vi "Teleop.vi"(10 "Match Info":T1={"Autonomous Elapsed Seconds"=0.0, "TeleOp Elapsed Seconds"=0.0, "Disabled Elapsed Seconds"=0.0, "Visited Autonomous"=FALSE, "Visited TeleOp"=FALSE, "Visited Disabled"=FALSE, "Autonomous Settings"={"Autonomous Style"=enum."Independent", "VI Refnum"=refnum}}, 11 "Call Context":T2) -> ()   [LabVIEW 2019]
doc: "This VI is called for each TeleOp packet received from the DS where the robot is not disabled. It is often used to read from the joysticks and update I/O or to update setpoints for timed control loops. It should complete and return within 20 milliseconds or it may miss DS packets."
uses:
  <vilib>/Rock Robotics/WPI/DriverStation/WPI_DriverStationDerivedRobotMode.ctl
  <vilib>/Rock Robotics/WPI/DriverStation/WPI_DriverStationMatch Info.ctl
  <vilib>/Rock Robotics/WPI/Solenoid/WPI_SolenoidValue.ctl
  <vilib>/Rock Robotics/WPI/ThirdParty/Phoenix-LabVIEW/Motor Controller/Controls/CTRE_Phoenix_MotorControl_ControlMode.ctl
  SubVi's/Joystick Organization/Joystick Global 6740.vi
  <vilib>/Rock Robotics/WPI/Solenoid/WPI_SolenoidSetEnum.vi
  <vilib>/Rock Robotics/WPI/ThirdParty/Phoenix-LabVIEW/Motor Controller/Get/CTRE_Phoenix_MotorController_GetSelectedSensorData.vi
  SubVi's/Global Conveyor.vi
panel:
  out "Color Count 2":dbl
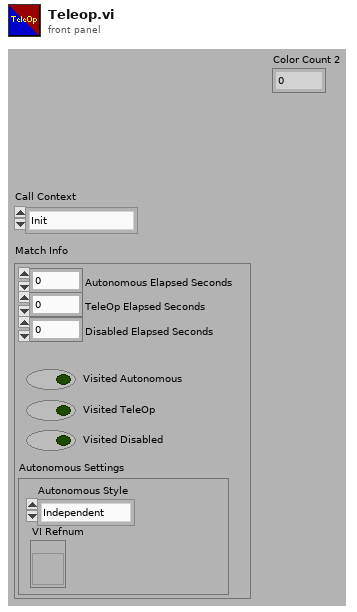
[diagram p1: front panel]
types:
  T1 = typedef "WPI_DriverStationMatch Info.ctl" = cluster{"Autonomous Elapsed Seconds":dbl, "TeleOp Elapsed Seconds":dbl, "Disabled Elapsed Seconds":dbl, "Visited Autonomous":bool, "Visited TeleOp":bool, "Visited Disabled":bool, "Autonomous Settings":cluster{"Autonomous Style":enum16{"Iterative", "Independent"}, "VI Refnum":refnum<vi>}}
  T2 = typedef "WPI_DriverStationDerivedRobotMode.ctl" = enum16{"Init", "Execute", "Stop"}
  T3 = typedef "WPI_SolenoidValue.ctl" = enum16{"Off", "On", "Forward", "Reverse"}
  T4 = typedef "WPI_MotorControlDeviceRef.ctl" = cluster{"DeviceStatus":errorcluster, "Type":T5, "PWM":cluster{"PWM Channel":T6, "DeadBand":T7}, "CAN":cluster{"Device Number":u8, "SetOutput VI Ref":variant, "GetOutput VI Ref":variant, "Enable VI Ref":variant, "Disable VI Ref":variant, "Data":variant}, "Invert":bool, "DIO PWM":cluster{"PWM \"Enable\" Channel":T6, "DIOChannel":T8, "PWM Rate":dbl}}
  T5 = typedef "WPI_MotorControlType.ctl" = enum16{"PWM", "CAN", "DIO PWM"}
  T6 = typedef "FPGA_DIOPWMChannel.ctl" = enum8{"PWM 0", "PWM 1", "PWM 2", "PWM 3", "PWM 4", "PWM 5", "PWM 6", "PWM 7", "PWM 8", "PWM 9", "PWM MXP 0", "PWM MXP 1", "PWM MXP 2", "PWM MXP 3", "PWM MXP 4", "PWM MXP 5", "PWM MXP 6", "PWM MXP 7", "PWM MXP 8", "PWM MXP 9", "Invalid"}
  T7 = typedef "WPI_PWMDeadband.ctl" = cluster{"Name":string, "maxPositivePwm":i32, "minPositivePwm":i32, "centerPwm":i32, "maxNegativePwm":i32, "minNegativePwm":i32, "angularRange":u16}
  T8 = typedef "FPGA_DIOChannel.ctl" = enum8{"DIO 0", "DIO 1", "DIO 2", "DIO 3", "DIO 4", "DIO 5", "DIO 6", "DIO 7", "DIO 8", "DIO 9", "DIO MXP 0", "DIO MXP 1", "DIO MXP 2", "DIO MXP 3", "DIO MXP 4", "DIO MXP 5", "DIO MXP 6", "DIO MXP 7", "DIO MXP 8", "DIO MXP 9", "DIO MXP 10", "DIO MXP 11", "DIO MXP 12", "DIO MXP 13", "DIO MXP 14", "DIO MXP 15", "SPI Port CS1", "SPI Port CS2", "SPI Port CS3", "SPI Port MISO", "SPI Port MOSI", "Invalid"}
  T9 = typedef "WPI_SolenoidDevRef.ctl" = cluster{"DevStatus":errorcluster, "Pneumatics Control Module":u8, "Forward Solenoid Channel":T10, "Reverse Solenoid Channel":T10}
  T10 = typedef "WPI_SolenoidChannel.ctl" = enum8{"Solenoid 0", "Solenoid 1", "Solenoid 2", "Solenoid 3", "Solenoid 4", "Solenoid 5", "Solenoid 6", "Solenoid 7", "Invalid"}
  T11 = typedef "Color Sensor V3 DevRef.ctl" = cluster{"I2CDevRef":T12}
  T12 = typedef "WPI_I2CDevRef.ctl" = cluster{"DevStatus":errorcluster, "Device Address":u8, "Handle":i32, "I2C Bus":T13}
  T13 = typedef "i2c_bus.ctl" = enum16{"I2C On-Board", "I2C MXP", "Invalid"}
  T14 = typedef "CTRE_Phoenix_MotorControl_ControlMode.ctl" = u16
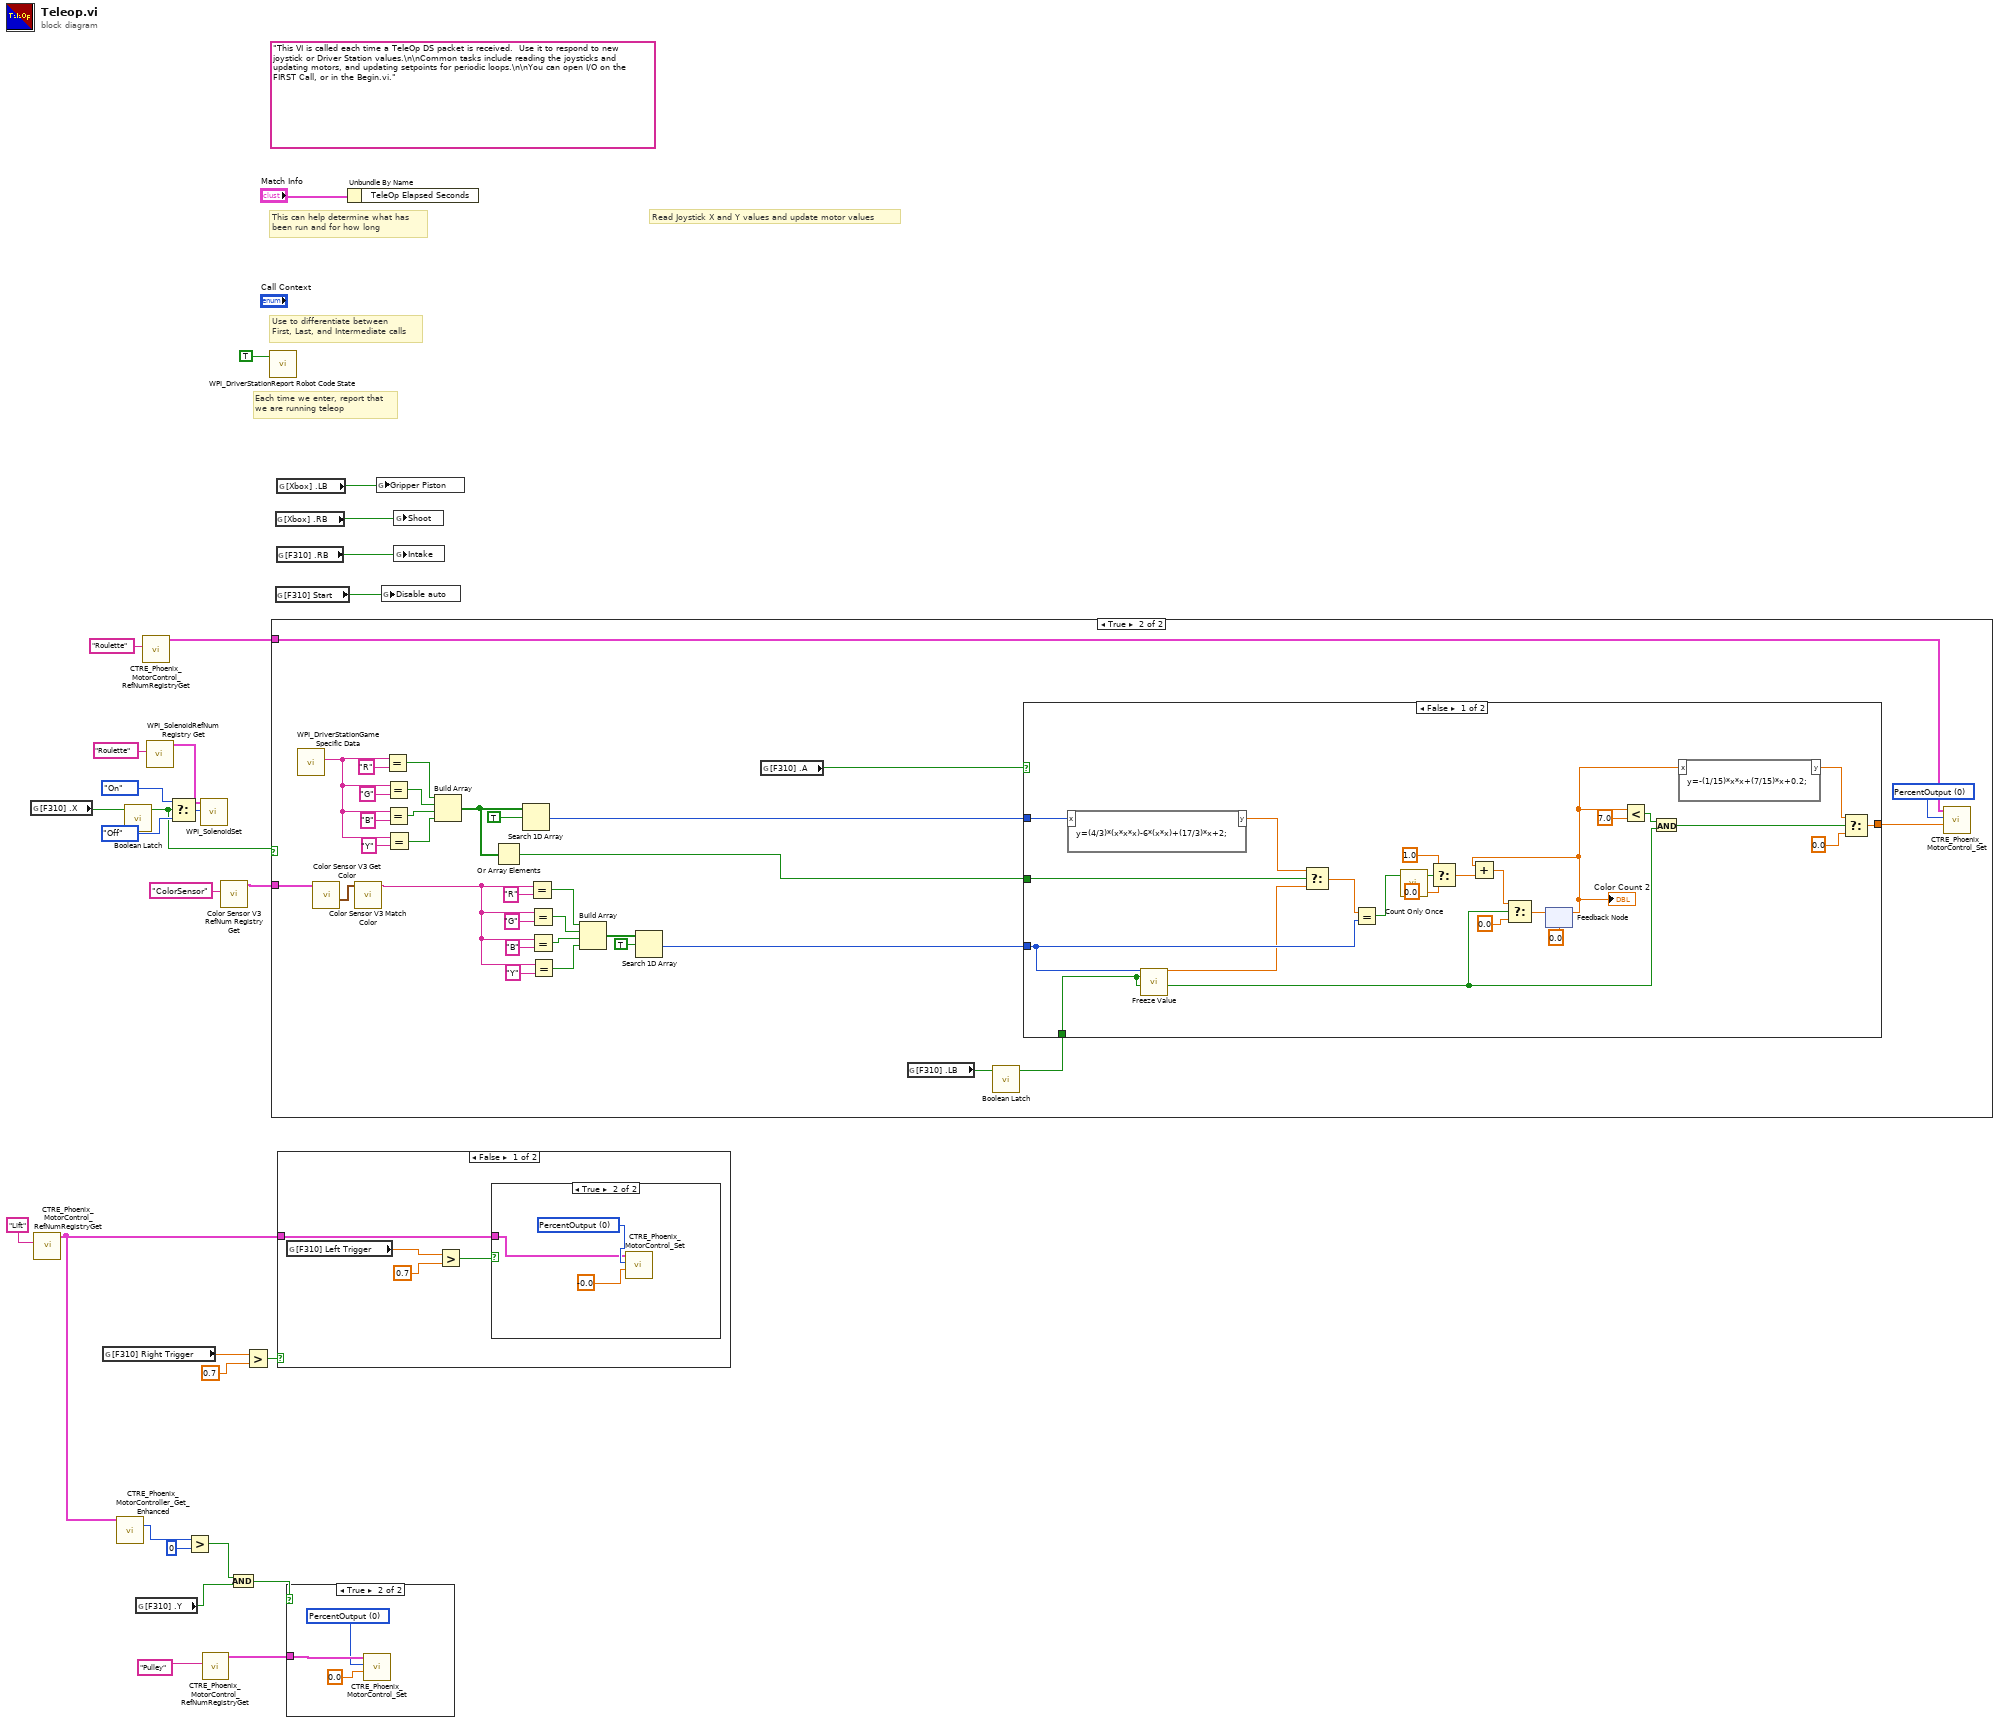
[diagram p0: block diagram]
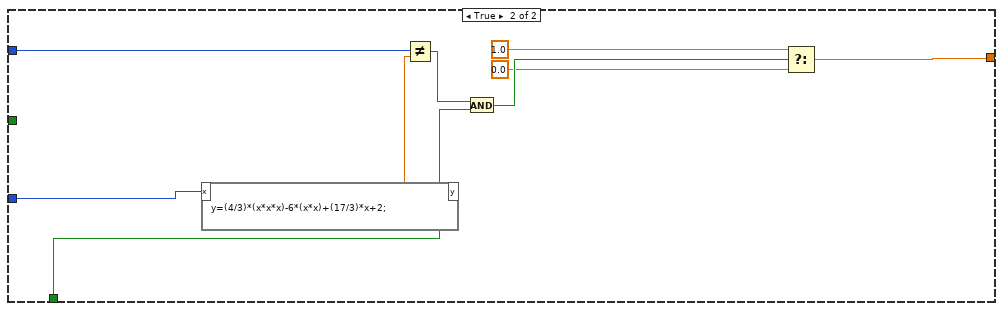
[diagram p3: hidden frame]
diagram:
  (unwired) "This VI is called each time a TeleOp DS packet is received.  Use it to respond to new joystick or Driver Station values.\n\nCommon tasks include reading the joysticks and updating motors, and updating setpoints for periodic loops.\n\nYou can open I/O on the FIRST Call, or in the Begin.vi."
  # "Each time we enter, report that\nwe are running teleop"
  # "Use to differentiate between\nFirst, Last, and Intermediate calls"
  # "This can help determine what has\nbeen run and for how long"
  # "Read Joystick X and Y values and update motor values"
  n1 = global read "Joystick Global 6740.vi" "[F310] .X"() -> (w13:bool)
  n2 = call <vilib>:"CTRE_Phoenix_MotorControl_RefNumRegistryGet.vi"("refnum name"="Lift") -> ("PhoenixMotorControlDevRef"=w23:T4)  [unwired: 9 in, 1 out]
  n3 = global read "Joystick Global 6740.vi" "[F310] Right Trigger"() -> (w27:dbl)
  n4 = call-poly <vilib>:"CTRE_Phoenix_MotorController_Get_Enhanced.vi"("PhoenixMotorControlDevRef"=w23) -> ("Position (Raw Sensor Units)"=w22:i32)  [unwired: 11 in, 3 out]
  n5 = call "Boolean Latch.vi"("Input"=w13) -> ("Output"=w7:bool)  [unwired: 26 in]
  n6 = global read "Joystick Global 6740.vi" "[F310] .Y"() -> (w19:bool)
  n7 = call <vilib>:"CTRE_Phoenix_MotorControl_RefNumRegistryGet.vi"("refnum name"="Roulette") -> ("PhoenixMotorControlDevRef"=w6:T4)  [unwired: 9 in, 1 out]
  n8 = call <vilib>:"WPI_SolenoidRefNum Registry Get.vi"("refnum name"="Roulette") -> ("SolenoidDevRef"=w14:T9)  [unwired: 9 in, 1 out]
  n9 = Select(t=WPI_SolenoidValue."On" ("Value"), s=w7, f=WPI_SolenoidValue."Off" ("Value")) -> (s? t:f=w10:T3)
  n10 = Greater?(x=w22, y=0) -> (0:w20:bool)
  n11 = call-poly <vilib>:"WPI_SolenoidSet.vi"("Value"=w10, "SolenoidDevRef"=w14) -> ()  [unwired: 8 in, 2 out]
  n12 = call <vilib>:"CTRE_Phoenix_MotorControl_RefNumRegistryGet.vi"("refnum name"="Pulley") -> ("PhoenixMotorControlDevRef"=w16:T4)  [unwired: 9 in, 1 out]
  n13 = call <vilib>:"Color Sensor V3 RefNum Registry Get.vi"("refnum name"="ColorSensor") -> ("ColorSensorDevRef"=w5:T11)  [unwired: 9 in, 1 out]
  n14 = And(x=w20, y=w19) -> (x .and. y?=w18:bool)
  n15 = Greater?(x=w27, y=0.7) -> (0:w25:bool)
  n16 = call <vilib>:"WPI_DriverStationReport Robot Code State.vi"("TeleOp"=TRUE ("Autonomous")) -> ()  [unwired: 10 in, 1 out]
  n17 = case shown="True" w7 {
    tunnel: w6 -> [_ w30]
    tunnel: w5 -> [_ w32]
    frame False {
    }
    frame True {
      w38 = T14 0 items=["PercentOutput"=0, "Position"=1, "Velocity"=2, "Current"=3, "Follower"=5, "MotionProfile"=6, "MotionMagic"=7, "MotionProfileArc"=10, "Disabled"=15] ("Control Mode")
      n18 = call <vilib>:"WPI_DriverStationGame Specific Data.vi"() -> ("Game Specific Data"=w35:string)  [unwired: 11 in]
      n19 = call <vilib>:"Color Sensor V3 Get Color.vi"("ColorSensorDevRef"=w32) -> ("Normalized Color"=w34:cluster{"R":dbl, "G":dbl, "B":dbl})  [unwired: 7 in, 3 out]
      n20 = call <vilib>:"Color Sensor V3 Match Color.vi"("Measured Color"=w34) -> ("Matched Color Name"=w33:string)  [unwired: 8 in, 2 out]
      n21 = Equal?(x=w35, y="R") -> (x = y?=w58:bool)
      n22 = Equal?(x=w35, y="G") -> (x = y?=w57:bool)
      n23 = Equal?(x=w35, y="B") -> (x = y?=w56:bool)
      n24 = Equal?(x=w35, y="Y") -> (x = y?=w55:bool)
      n25 = Build Array(w58, w57, w56, w55) -> (w42:bool[])
      n26 = Or Array Elements(Boolean array=w42) -> (logical OR=w40:bool)
      n27 = Search 1D Array(1D array=w42, element=TRUE) -> (index of element=w41:i32)  [unwired: 1 in]
      n28 = Equal?(x=w33, y="R") -> (x = y?=w52:bool)
      n29 = Equal?(x=w33, y="G") -> (x = y?=w51:bool)
      n30 = Equal?(x=w33, y="B") -> (x = y?=w50:bool)
      n31 = Equal?(x=w33, y="Y") -> (x = y?=w49:bool)
      n32 = Build Array(w52, w51, w50, w49) -> (w53:bool[])
      n33 = Search 1D Array(1D array=w53, element=TRUE) -> (index of element=w39:i32)  [unwired: 1 in]
      n34 = global read "Joystick Global 6740.vi" "[F310] .A"() -> (w36:bool)
      n35 = global read "Joystick Global 6740.vi" "[F310] .LB"() -> (w31:bool)
      n36 = call "Boolean Latch.vi"("Input"=w31) -> ("Output"=w43:bool)  [unwired: 26 in]
      n37 = case shown="False" w36 {
        tunnel: w41 -> [w85 w94]
        tunnel: w43 -> [w68 w92]
        tunnel: [w70 w89] -> w37
        tunnel: w40 -> [w67 _]
        tunnel: w39 -> [w84 w91]
        frame False {
          n38 = formula code="y=(4/3)*(x*x*x)-6*(x*x)+(17/3)*x+2;"("x"=w85) -> ("y"=w78:dbl)
          n39 = call "Freeze Value.vi"("Input"=w84, "Freeze Value"=w68) -> ("Output"=w83:dbl)  [unwired: 25 in]
          n40 = Select(t=w78, s=w67, f=w83) -> (s? t:f=w77:dbl)
          n41 = Equal?(x=w77, y=w84) -> (x = y?=w64:bool)
          n42 = call "Count Only Once.vi"("InValue"=w64) -> ("Result"=w63:bool)  [unwired: 26 in]
          n43 = Select(t=1.0, s=w63, f=0.0) -> (s? t:f=w76:dbl)
          n44 = feedback #1(0.0) -> (w65:dbl)
          "Color Count 2" <- w65
          n45 = Add(x=w65, y=w76) -> (x+y=w74:dbl)
          n46 = Select(t=w74, s=w68, f=0.0) -> (s? t:f=w75:dbl)
          n47 = feedback-in #1(w75) -> ()
          n48 = Less?(x=w65, y=7.0) -> (x < y?=w72:bool)
          n49 = And(x=w72, y=w68) -> (x .and. y?=w71:bool)
          n50 = formula code="y=-(1/15)*x*x+(7/15)*x+0.2;"("x"=w65) -> ("y"=w66:dbl)
          n51 = Select(t=w66, s=w71, f=0.0) -> (s? t:f=w70:dbl)
        }
        frame True {
          n52 = formula code="y=(4/3)*(x*x*x)-6*(x*x)+(17/3)*x+2;"("x"=w91) -> ("y"=w90:dbl)
          n53 = Not Equal?(x=w94, y=w90) -> (x != y?=w93:bool)
          n54 = And(x=w93, y=w92) -> (x .and. y?=w88:bool)
          n55 = Select(t=1.0, s=w88, f=0.0) -> (s? t:f=w89:dbl)
        }
      }
      n56 = call <vilib>:"CTRE_Phoenix_MotorControl_Set.vi"("Output"=w37, "Control Mode"=w38, "PhoenixMotorControlDevRef"=w30) -> ()  [unwired: 7 in, 2 out]
    }
  }
  n57 = global read "Joystick Global 6740.vi" "[Xbox] .RB"() -> (w4:bool)
  n58 = global read "Joystick Global 6740.vi" "[F310] Start"() -> (w1:bool)
  n59 = global read "Joystick Global 6740.vi" "[F310] .RB"() -> (w3:bool)
  n60 = global read "Joystick Global 6740.vi" "[Xbox] .LB"() -> (w2:bool)
  n61 = case shown="False" w25 {
    tunnel: w23 -> [w95 _]
    frame False {
      n62 = global read "Joystick Global 6740.vi" "[F310] Left Trigger"() -> (w98:dbl)
      n63 = Greater?(x=w98, y=0.7) -> (0:w96:bool)
      n64 = case shown="True" w96 {
        tunnel: w95 -> [_ w99]
        frame False {
        }
        frame True {
          w100 = T14 0 items=["PercentOutput"=0, "Position"=1, "Velocity"=2, "Current"=3, "Follower"=5, "MotionProfile"=6, "MotionMagic"=7, "MotionProfileArc"=10, "Disabled"=15] ("Control Mode")
          n65 = call <vilib>:"CTRE_Phoenix_MotorControl_Set.vi"("Output"=-0.0, "Control Mode"=w100, "PhoenixMotorControlDevRef"=w99) -> ()  [unwired: 7 in, 2 out]
        }
      }
    }
    frame True {
    }
  }
  n66 = case shown="True" w18 {
    tunnel: w16 -> [_ w104]
    frame False {
    }
    frame True {
      w103 = T14 0 items=["PercentOutput"=0, "Position"=1, "Velocity"=2, "Current"=3, "Follower"=5, "MotionProfile"=6, "MotionMagic"=7, "MotionProfileArc"=10, "Disabled"=15] ("Control Mode")
      n67 = call <vilib>:"CTRE_Phoenix_MotorControl_Set.vi"("Output"=0.0, "Control Mode"=w103, "PhoenixMotorControlDevRef"=w104) -> ()  [unwired: 7 in, 2 out]
    }
  }
  n68 = Unbundle By Name("Match Info") -> ()  [unwired: 1 out]
  n69 = global write "Global Conveyor.vi" "Gripper Piston"(w2) -> ()
  n70 = global write "Global Conveyor.vi" "Disable auto"(w1) -> ()
  n71 = global write "Global Conveyor.vi" "Shoot"(w4) -> ()
  n72 = global write "Global Conveyor.vi" "Intake"(w3) -> ()
